vi "Indexing objective waveform.vi"(1 "Waveform":waveform(dbl), 2 "Window size for layer index (ms)":dbl, 3 "Backward Time (s)":dbl, 4 "Z stack backward 采样信息":cluster{"采样率":dbl, "采样数":dbl}, 5 "Z stack acquisition 采样信息":cluster{"采样率":dbl, "采样数":dbl}, 6 "Steps per Volume":dbl) -> (0 "digital waveform":digitalwaveform(waveform))   [LabVIEW 2018]
uses:
  <vilib>/measure/mascope.llb/Transition Measurements 1 chan.vi
  <vilib>/Waveform/WDTOps.llb/WDT Append Waveforms DBL.vi
  <vilib>/Waveform/DWDTOps.llb/DWDT Analog to Digital.vi
  <vilib>/measure/NI_MABase.lvlib
  <vilib>/measure/NI_MAPro.lvlib
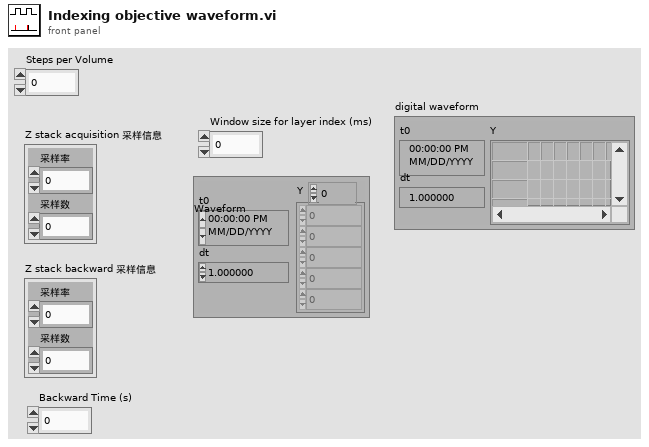
[diagram p1: front panel]
types:
  T1 = cluster{"high ref level":dbl, "mid ref level":dbl, "low ref level":dbl, "ref units":u16}
  T2 = cluster{"start time":dbl, "end time":dbl, "ref levels":cluster{"high ref level":dbl, "mid ref level":dbl, "low ref level":dbl, "ref units":u16}}
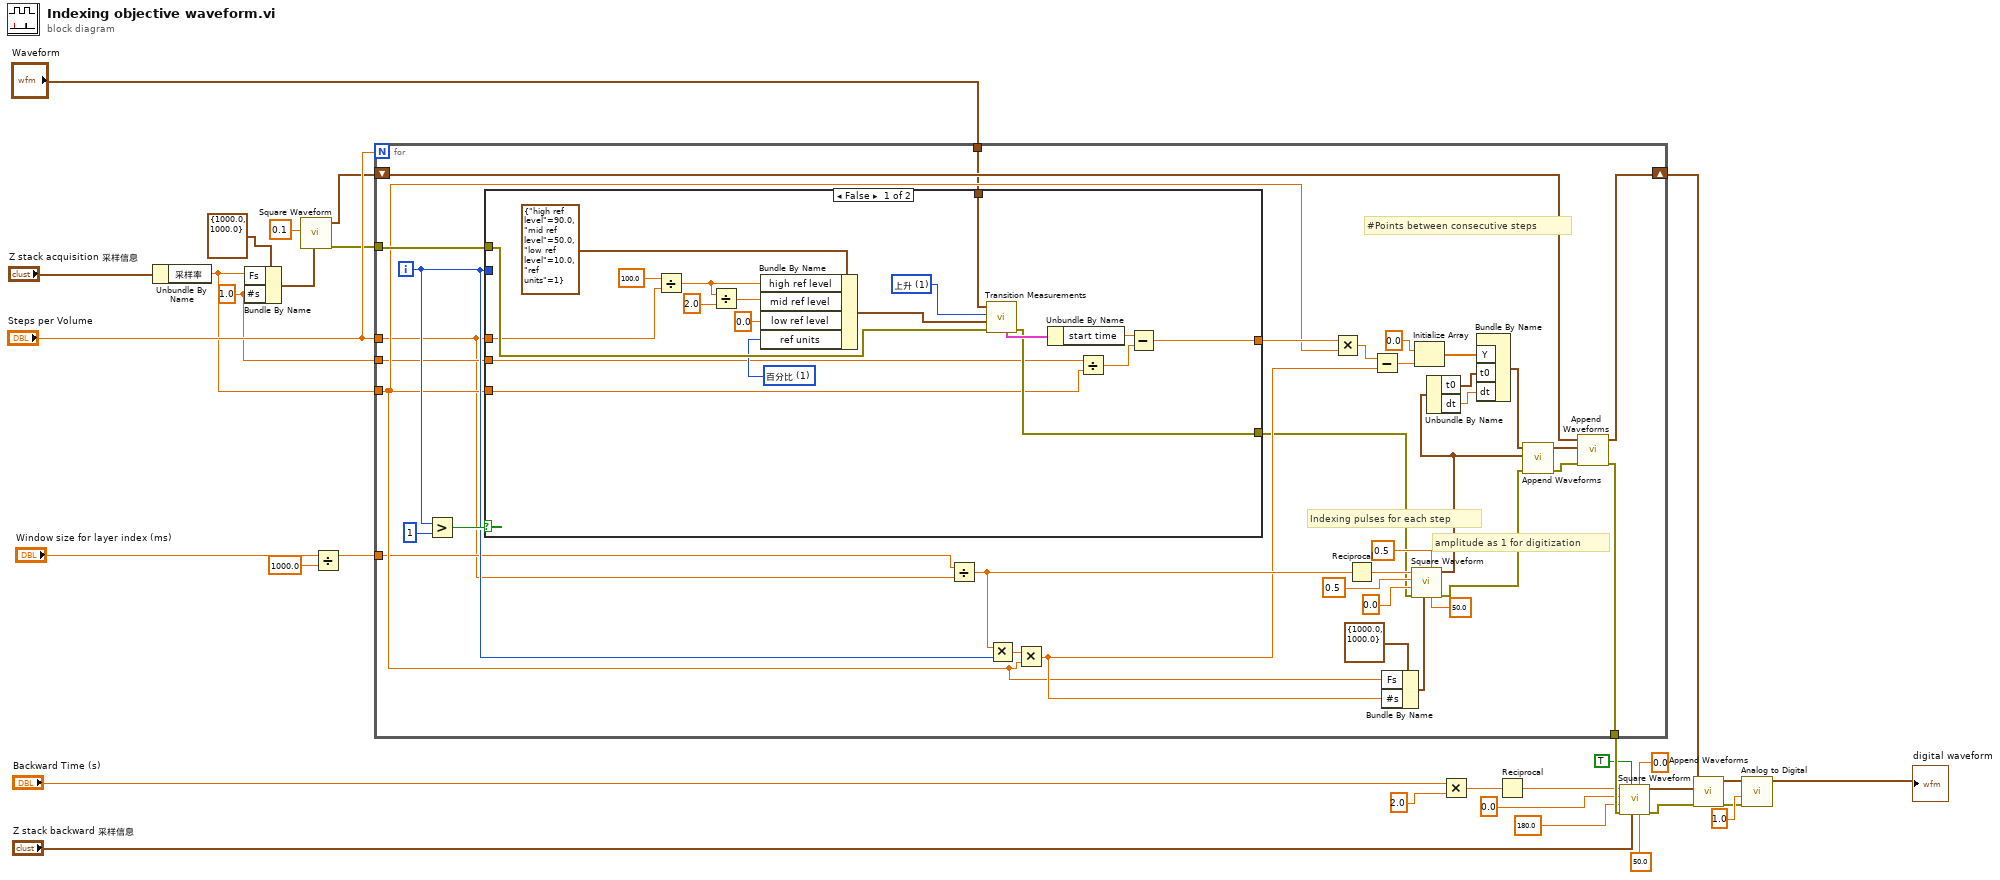
[diagram p0: block diagram]
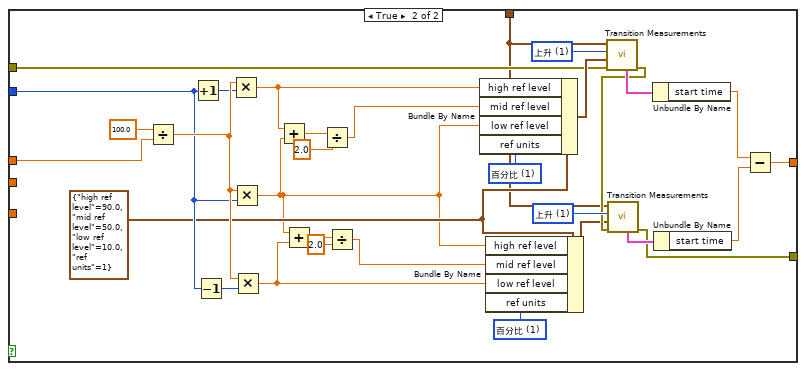
[diagram p2: hidden frame]
diagram:
  w26 = 1.0 ("#s")
  n1 = Unbundle By Name("Z stack acquisition 采样信息") -> ("采样率"=w27:dbl)
  n2 = Bundle By Name(cluster=cluster{"Fs":dbl, "#s":dbl} {"Fs"=1000.0, "#s"=1000.0} ("sampling info"), "Fs"=w27, "#s"=w26) -> (w19:cluster{"Fs":dbl, "#s":dbl})
  n3 = call <vilib>:"Square Waveform.vi"("sampling info"=w19, "amplitude"=0.1) -> ("error out"=w22:errorcluster, "signal out"=w20:waveform(dbl))  [unwired: 8 in]
  n4 = Divide(x="Window size for layer index (ms)", y=1000.0) -> (x/y=w6:dbl)
  n5 = for {
    N: "Steps per Volume" -> [_]
    shift-right: [w45] -> w3
    shift-left: w20 -> [w46]
    tunnel: [w41] -> w21
    tunnel: w22 -> [w40]
    tunnel: w26 -> [w34]
    tunnel: w27 -> [w39]
    tunnel: "Waveform" -> [w35]
    tunnel: "Steps per Volume" -> [w32]
    tunnel: w6 -> [w33]
    i -> [w55]
    # "amplitude as 1 for digitization"
    # "Indexing pulses for each step"
    # "#Points between consecutive steps"
    n6 = Greater?(x=w55, y=1) -> (0:w56:bool)
    n7 = case shown="False" w56 {
      tunnel: w35 -> [w85 w87]
      tunnel: w55 -> [_ w110]
      tunnel: [w71 w103] -> w53
      tunnel: [w77 w101] -> w44
      tunnel: w40 -> [w78 w100]
      tunnel: w34 -> [w69 _]
      tunnel: w39 -> [w68 _]
      tunnel: w32 -> [w67 w86]
      frame False {
        w76 = u16 1 items=["绝对", "百分比"] ("ref units")
        w84 = u16 1 items=["下降", "上升"] ("polarity (rising)")
        n8 = Divide(x=100.0, y=w67) -> (x/y=w74:dbl)
        n9 = Divide(x=w74, y=2.0) -> (x/y=w75:dbl)
        n10 = Bundle By Name(cluster=T1 {"high ref level"=90.0, "mid ref level"=50.0, "low ref level"=10.0, "ref units"=1} ("reference levels 2"), "high ref level"=w74, "mid ref level"=w75, "low ref level"=0.0, "ref units"=w76) -> (w82:T1)
        n11 = call-poly <vilib>:"Transition Measurements.vi"("error in (no error)"=w78, "reference levels"=w82, "polarity (rising)"=w84, "signal in"=w85) -> ("error out"=w77:errorcluster, "measurement info"=w79:T2)  [unwired: 2 in, 4 out]
        n12 = Unbundle By Name(w79) -> ("start time"=w72:dbl)
        n13 = Divide(x=w69, y=w68) -> (x/y=w70:dbl)
        n14 = Subtract(x=w72, y=w70) -> (x-y=w71:dbl)
      }
      frame True {
        w98 = u16 1 items=["绝对", "百分比"] ("ref units")
        w99 = u16 1 items=["绝对", "百分比"] ("ref units 2")
        w106 = T1 {"high ref level"=90.0, "mid ref level"=50.0, "low ref level"=10.0, "ref units"=1} ("reference levels")
        w114 = u16 1 items=["下降", "上升"] ("polarity (rising)")
        w116 = u16 1 items=["下降", "上升"] ("polarity (rising)")
        n15 = Divide(x=100.0, y=w86) -> (x/y=w111:dbl)
        n16 = Increment(x=w110) -> (x+1=w109:i32)
        n17 = Decrement(x=w110) -> (x-1=w108:i32)
        n18 = Multiply(x=w111, y=w109) -> (x*y=w90:dbl)
        n19 = Multiply(x=w111, y=w110) -> (x*y=w88:dbl)
        n20 = Multiply(x=w111, y=w108) -> (x*y=w89:dbl)
        n21 = Add(x=w90, y=w88) -> (x+y=w96:dbl)
        n22 = Add(x=w88, y=w89) -> (x+y=w94:dbl)
        n23 = Divide(x=w96, y=2.0) -> (x/y=w95:dbl)
        n24 = Divide(x=w94, y=2.0) -> (x/y=w93:dbl)
        n25 = Bundle By Name(cluster=w106, "high ref level"=w90, "mid ref level"=w95, "low ref level"=w88, "ref units"=w98) -> (w107:T1)
        n26 = Bundle By Name(cluster=w106, "high ref level"=w88, "mid ref level"=w93, "low ref level"=w89, "ref units"=w99) -> (w97:T1)
        n27 = call-poly <vilib>:"Transition Measurements.vi"("error in (no error)"=w100, "reference levels"=w107, "polarity (rising)"=w114, "signal in"=w87) -> ("error out"=w102:errorcluster, "measurement info"=w112:T2)  [unwired: 2 in, 4 out]
        n28 = call-poly <vilib>:"Transition Measurements.vi"("error in (no error)"=w102, "reference levels"=w97, "polarity (rising)"=w116, "signal in"=w87) -> ("error out"=w101:errorcluster, "measurement info"=w115:T2)  [unwired: 2 in, 4 out]
        n29 = Unbundle By Name(w112) -> ("start time"=w105:dbl)
        n30 = Unbundle By Name(w115) -> ("start time"=w104:dbl)
        n31 = Subtract(x=w105, y=w104) -> (x-y=w103:dbl)
      }
    }
    n32 = Divide(x=w33, y=w32) -> (x/y=w61:dbl)
    n33 = Multiply(x=w61, y=w55) -> (x*y=w60:dbl)
    n34 = Multiply(x=w60, y=w39) -> (x*y=w52:dbl)
    n35 = Multiply(x=w53, y=w39) -> (x*y=w54:dbl)
    n36 = Reciprocal(x=w61) -> (1/x=w66:dbl)
    n37 = Subtract(x=w54, y=w52) -> (x-y=w51:dbl)
    n38 = Bundle By Name(cluster=cluster{"Fs":dbl, "#s":dbl} {"Fs"=1000.0, "#s"=1000.0} ("sampling info"), "Fs"=w39, "#s"=w52) -> (w58:cluster{"Fs":dbl, "#s":dbl})
    n39 = call <vilib>:"Square Waveform.vi"("duty cycle (%)"=50.0, "offset"=0.5, "sampling info"=w58, "error in (no error)"=w44, "phase"=0.0, "amplitude"=0.5, "frequency"=w66) -> ("error out"=w43:errorcluster, "signal out"=w36:waveform(dbl))  [unwired: 3 in]
    n40 = Initialize Array(0.0 ("元素"), w51) -> (w49:dbl[])
    n41 = Unbundle By Name(w36) -> ("t0"=w38:timestamp, "dt"=w37:dbl)
    n42 = Bundle By Name("Y"=w49, "t0"=w38, "dt"=w37) -> (w48:waveform(dbl))  [unwired: 1 in]
    n43 = call-poly <vilib>:"Append Waveforms.vi"("error in (no error)"=w43, "waveform B"=w36, "waveform A"=w48) -> ("error out"=w42:errorcluster, "waveform out"=w47:waveform(dbl))  [unwired: 7 in]
    n44 = call-poly <vilib>:"Append Waveforms.vi"("error in (no error)"=w42, "waveform B"=w47, "waveform A"=w46) -> ("error out"=w41:errorcluster, "waveform out"=w45:waveform(dbl))  [unwired: 7 in]
  }
  n45 = Multiply(x="Backward Time (s)", y=2.0) -> (x*y=w9:dbl)
  n46 = Reciprocal(x=w9) -> (1/x=w10:dbl)
  n47 = call <vilib>:"Square Waveform.vi"("duty cycle (%)"=50.0, "offset"=0.0, "sampling info"="Z stack backward 采样信息", "reset signal"=TRUE, "error in (no error)"=w21, "phase"=180.0, "amplitude"=0.0, "frequency"=w10) -> ("error out"=w14:errorcluster, "signal out"=w2:waveform(dbl))  [unwired: 2 in]
  n48 = call-poly <vilib>:"Append Waveforms.vi"("error in (no error)"=w14, "waveform B"=w2, "waveform A"=w3) -> ("error out"=w23:errorcluster, "waveform out"=w4:waveform(dbl))  [unwired: 7 in]
  n49 = call-poly <vilib>:"Analog to Digital.vi"("error in (no error)"=w23, "full-scale range (pk-pk)"=1.0, "analog waveform"=w4) -> ("digital waveform"=→"digital waveform":digitalwaveform)  [unwired: 5 in, 3 out]
